vi "AI Base Close.vi"(8 "error in":errorcluster, 10 "Http Refnum in":T1, 11 "Python Refnum in":refnum<k35>) -> (0 "error out":errorcluster)   [LabVIEW 2023, in "LabVIEW AI Base.lvlib"]
uses:
  <vilib>/httpClient/ClientHandle.ctl
  LabVIEW AI Base.lvlib
  <vilib>/httpClient/LabVIEWHTTPClient.lvlib
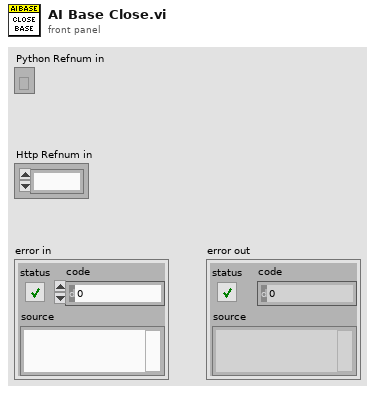
[diagram p1: front panel]
types:
  T1 = typedef "LabVIEWHTTPClient.lvlib/ClientHandle.ctl" = refnum<k1>
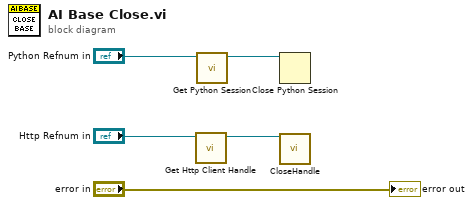
[diagram p0: block diagram]
diagram:
  n1 = call "Get Http Client Handle.vi"("Refnum in"="Http Refnum in") -> ("Refnum out"=w3:T1)  [unwired: 10 in]
  n2 = call "Get Python Session.vi"("Python Session in"="Python Refnum in") -> ("Python Session out"=w2:refnum<k35>)  [unwired: 10 in]
  n3 = Close Python Session(session in=w2) -> ()  [unwired: 1 in, 1 out]
  n4 = call <vilib>:"CloseHandle.vi"("client handle"=w3) -> ()  [unwired: 14 in, 1 out]
  "error out" <- "error in"
